vi "Moment Score.vi"(11 "Moment Factor":dbl) -> (3 "Score":dbl)   [LabVIEW 2017]
doc: "Calculate a score based on area and convex hull area. Convex hull area fills holes and convex areas of the shape. It is equivalent to putting a rubber band around the shape and computing the area enclosed by the band."
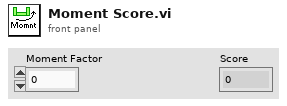
[diagram p1: front panel]
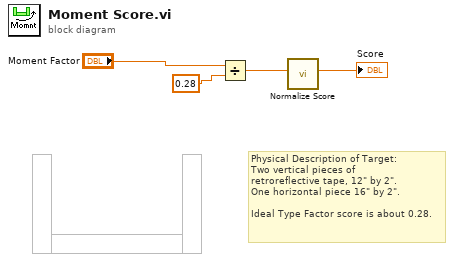
[diagram p0: block diagram]
diagram:
  # "Physical Description of Target:\nTwo vertical pieces of\nretroreflective tape, 12\" by 2\".\nOne horizontal piece 16\" by 2\".\n\nIdeal Type Factor score is about 0.28."
  n1 = Divide(x="Moment Factor", y=0.28 ("length")) -> (x/y=w3:dbl)
  n2 = call "Normalize Score.vi"("Value"=w3) -> ("Score"=→"Score":dbl)  [unwired: 10 in]
